vi "TL Motor StartCtrl.vi"() -> ()   [LabVIEW 2021]
doc: "Shows how to Start a motor control."
panel:
  in  "MG17Motor":refnum<k7>(container)
  in  "Stop":bool
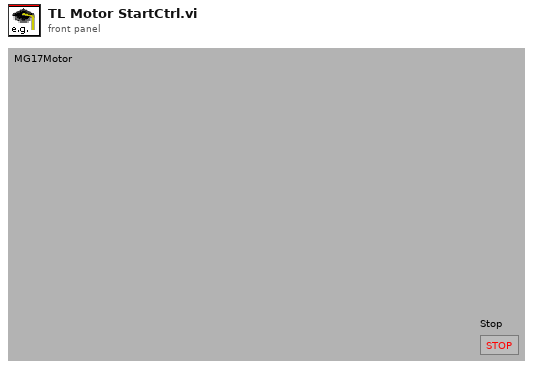
[diagram p1: front panel]
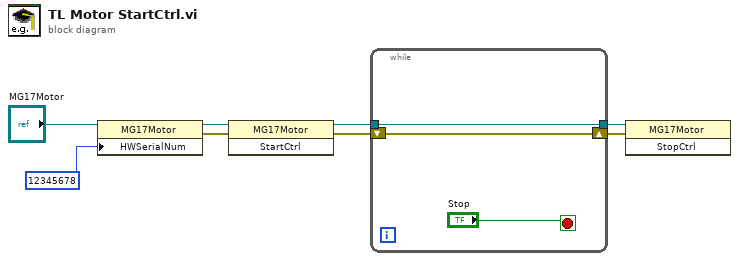
[diagram p0: block diagram]
diagram:
  n1 = property class="MG17Motor"(reference="MG17Motor", "HWSerialNum"=12345678) -> (reference out=w4:refnum<k7>, error out=w5:errorcluster)  [unwired: 1 in]
  n2 = invoke class="MG17Motor" method="StartCtrl"(reference=w4, error in=w5) -> (reference out=w3:refnum<k7>, error out=w2:errorcluster)  [unwired: 1 in, 1 out]
  n3 = while {
    shift-left: w2 -> [w10]
    shift-right: [w10] -> w8
    tunnel: w3 -> [w9]
    tunnel: [w9] -> w6
    stop <- "Stop" stop-if-true
  }
  n4 = invoke class="MG17Motor" method="StopCtrl"(reference=w6, error in=w8) -> ()  [unwired: 1 in, 3 out]
